vi "USB2XXXGPIOTest.vi"() -> ()   [LabVIEW 2010]
uses:
  PublicFiles/USB2XXX.dll
panel:
  out "P15":bool
  out "P14":bool
  out "P13":bool
  out "P12":bool
  out "P11":bool
  out "P10":bool
  out "P9":bool
  out "P8":bool
  in  "P7":bool
  in  "P6":bool
  in  "P5":bool
  in  "P4":bool
  in  "P3":bool
  in  "P2":bool
  in  "P1":bool
  in  "P0":bool
  in  "Device Index":i32(ring) items=["0", "1", "2", "3", "4", "5"]
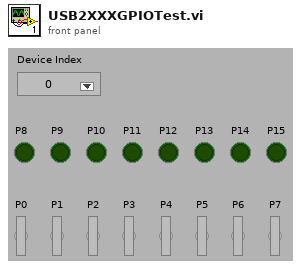
[diagram p1: front panel]
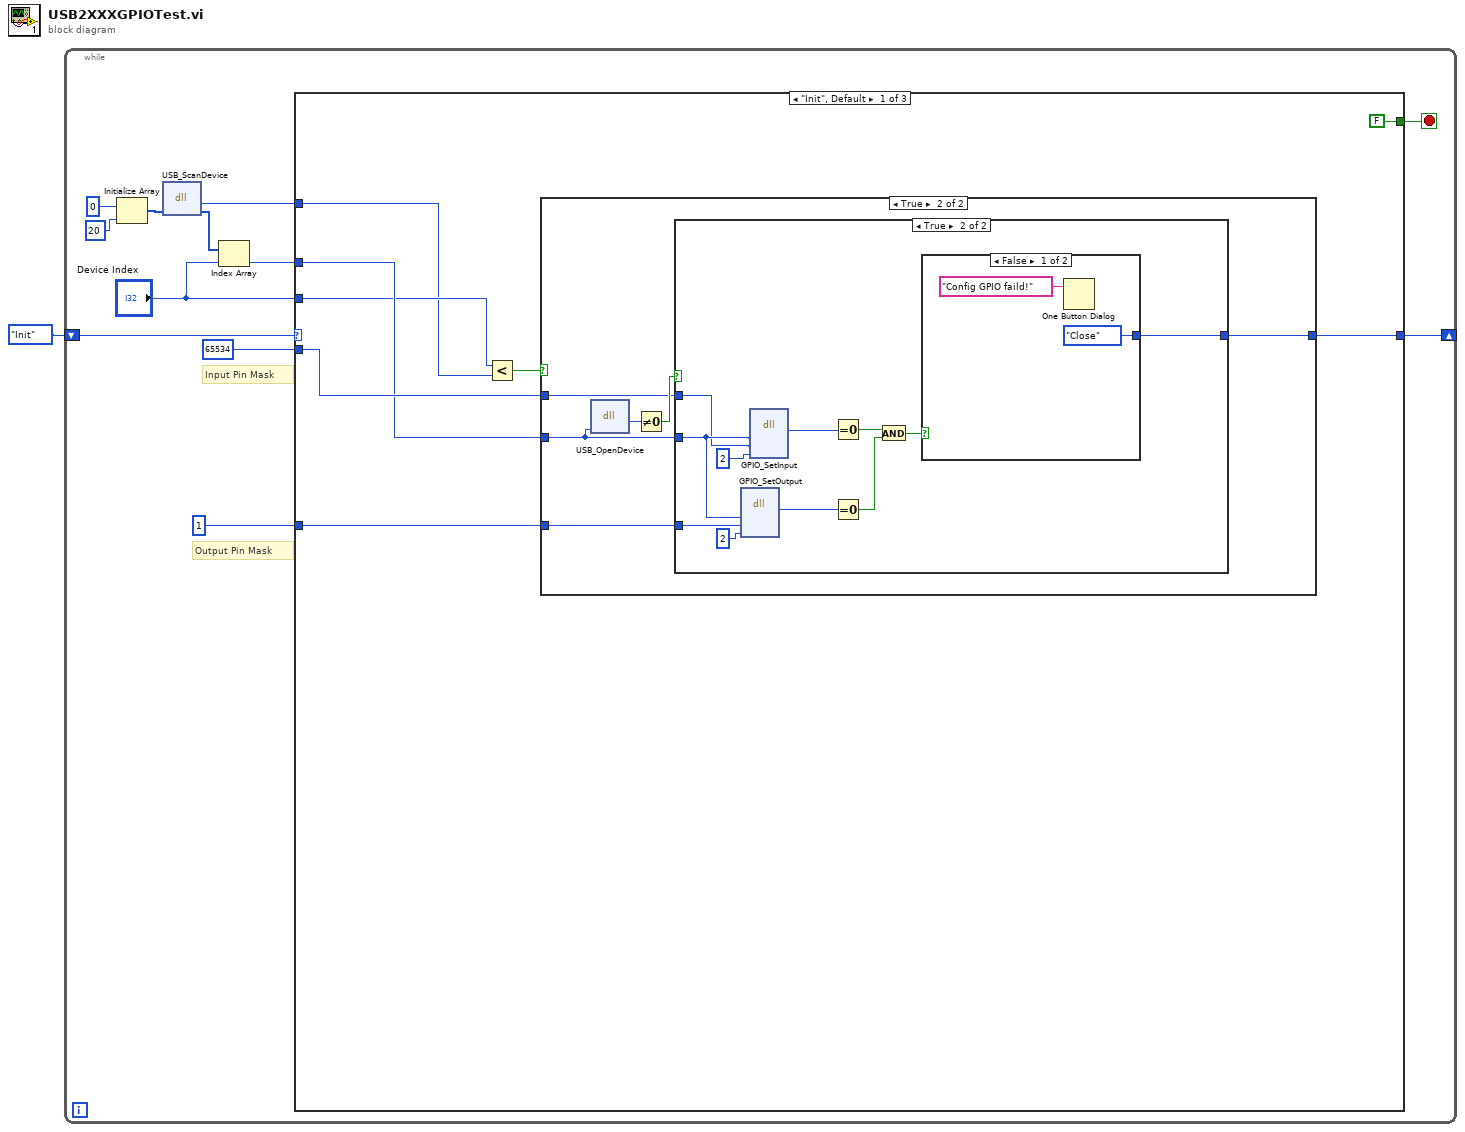
[diagram p0: block diagram]
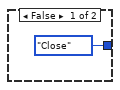
[diagram p2: hidden frame]
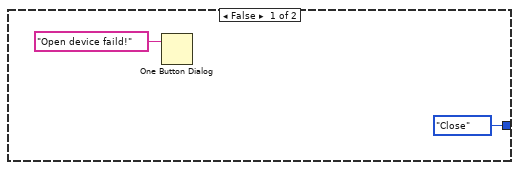
[diagram p3: hidden frame]
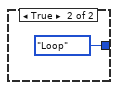
[diagram p4: hidden frame]
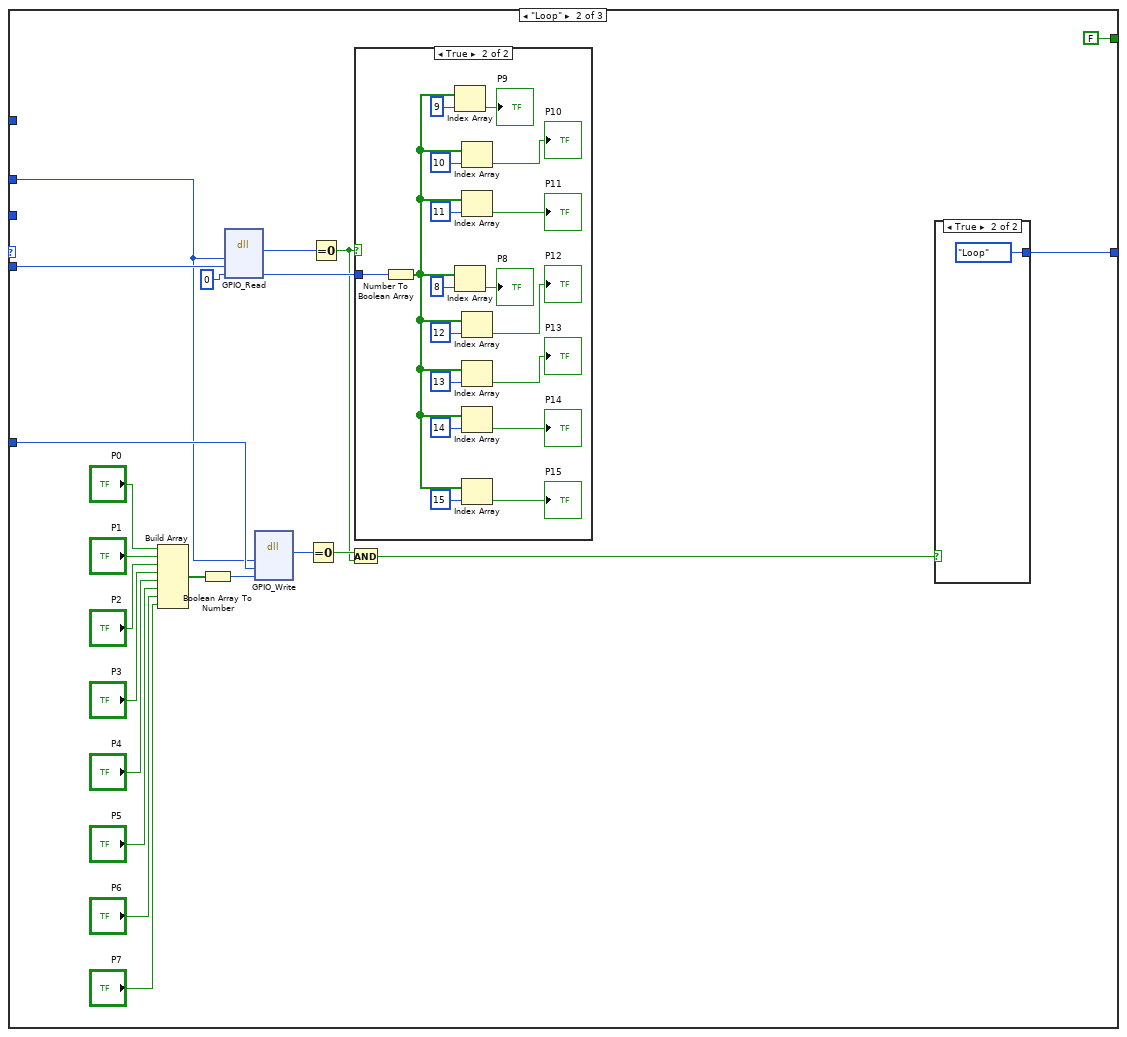
[diagram p5: hidden frame]
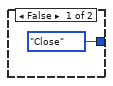
[diagram p6: hidden frame]
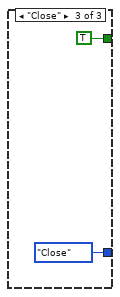
[diagram p8: hidden frame]
diagram:
  n1 = while {
    shift-right: [w12] -> _
    shift-left: enum16{"Init", "Loop", "Close"}."Init" ("Enum") -> [w13]
    stop <- w11 stop-if-true
    # "Output Pin Mask"
    # "Input Pin Mask"
    n2 = Initialize Array(0, 20 ("dimension size")) -> (w8:i32[])
    n3 = dll-call lib="E:/OtherWork/STM32/USB2XXX_Example/trunk/Labview/PublicFiles/USB2XXX.*" fn="USB_ScanDevice"("pDevNum"=w8) -> ("return type"=w4:i32, "pDevNum"=w5:i32[])  [unwired: 3 in, 2 out]
    n4 = Index Array(array=w5, index="Device Index") -> (element=w3:i32)
    n5 = case shown="\"Init\", Default" w13 {
      tunnel: [w20 w46 enum16{"Init", "Loop", "Close"}."Close" ("Enum")] -> w12
      tunnel: u32 65534 -> [w17 w54 _]
      tunnel: [FALSE FALSE TRUE] -> w11
      tunnel: u32 1 -> [w18 w56 _]
      tunnel: w4 -> [w14 _ _]
      tunnel: w3 -> [w16 w45 _]
      tunnel: "Device Index" -> [w15 _ _]
      frame "Init", Default {
        n6 = Less?(x=w15, y=w14) -> (x < y?=w21:bool)
        n7 = case shown="True" w21 {
          tunnel: w16 -> [_ w26]
          tunnel: [enum16{"Init", "Loop", "Close"}."Close" ("Enum") w25] -> w20
          tunnel: w18 -> [_ w24]
          tunnel: w17 -> [_ w23]
          frame False {
          }
          frame True {
            n8 = dll-call lib="E:/OtherWork/STM32/USB2XXX_Example/trunk/Labview/PublicFiles/USB2XXX.*" fn="USB_OpenDevice"("DevIndex"=w26) -> (w28:u8)  [unwired: 4 in, 2 out]
            n9 = Not Equal To 0?(x=w28) -> (x != 0?=w27:bool)
            n10 = case shown="True" w27 {
              tunnel: w26 -> [_ w34]
              tunnel: [enum16{"Init", "Loop", "Close"}."Close" ("Enum") w41] -> w25
              tunnel: w24 -> [_ w40]
              tunnel: w23 -> [_ w33]
              frame False {
                n11 = One Button Dialog(message="Open device faild!") -> ()  [unwired: 1 in, 1 out]
              }
              frame True {
                n12 = dll-call lib="E:/OtherWork/STM32/USB2XXX_Example/trunk/Labview/PublicFiles/USB2XXX.*" fn="GPIO_SetOutput"("DevIndex"=w34, "PinMask"=w40, "PuPd"=u8 2) -> (w38:i32)  [unwired: 6 in, 2 out]
                n13 = dll-call lib="E:/OtherWork/STM32/USB2XXX_Example/trunk/Labview/PublicFiles/USB2XXX.*" fn="GPIO_SetInput"("DevHandle"=w34, "PinMask"=w33, "PuPd"=u8 2) -> (w31:i32)  [unwired: 6 in, 2 out]
                n14 = Equal To 0?(x=w31) -> (x = 0?=w37:bool)
                n15 = Equal To 0?(x=w38) -> (x = 0?=w36:bool)
                n16 = And(x=w37, y=w36) -> (x .and. y?=w35:bool)
                n17 = case shown="False" w35 {
                  tunnel: [enum16{"Init", "Loop", "Close"}."Close" ("Enum") enum16{"Init", "Loop", "Close"}."Loop" ("Enum")] -> w41
                  frame False {
                    n18 = One Button Dialog(message="Config GPIO faild!") -> ()  [unwired: 1 in, 1 out]
                  }
                  frame True {
                  }
                }
              }
            }
          }
        }
      }
      frame "Loop" {
        n19 = Build Array("P0", "P1", "P2", "P3", "P4", "P5", "P6", "P7") -> (w57:bool[])
        n20 = Boolean Array To Number(Boolean array=w57) -> (number=w55:u32)
        n21 = dll-call lib="E:/OtherWork/STM32/USB2XXX_Example/trunk/Labview/PublicFiles/USB2XXX.*" fn="GPIO_Read"("DevIndex"=w45, "PinMask"=w54, "pPinValue"=u32 0) -> (w52:i32, "pPinValue"=w51:u32)  [unwired: 5 in, 2 out]
        n22 = dll-call lib="E:/OtherWork/STM32/USB2XXX_Example/trunk/Labview/PublicFiles/USB2XXX.*" fn="GPIO_Write"("DevIndex"=w45, "PinMask"=w56, "PinValue"=w55) -> (w50:i32)  [unwired: 6 in, 2 out]
        n23 = Equal To 0?(x=w50) -> (x = 0?=w49:bool)
        n24 = Equal To 0?(x=w52) -> (x = 0?=w48:bool)
        n25 = And(x=w49, y=w48) -> (x .and. y?=w47:bool)
        n26 = case shown="True" w48 {
          tunnel: w51 -> [_ w86]
          frame False {
          }
          frame True {
            n27 = Number To Boolean Array(number=w86) -> (Boolean array=w76:bool[])
            n28 = Index Array(array=w76, index=9) -> (element=→"P9":bool)
            n29 = Index Array(array=w76, index=8) -> (element=→"P8":bool)
            n30 = Index Array(array=w76, index=10) -> (element=→"P10":bool)
            n31 = Index Array(array=w76, index=11) -> (element=→"P11":bool)
            n32 = Index Array(array=w76, index=12) -> (element=→"P12":bool)
            n33 = Index Array(array=w76, index=13) -> (element=→"P13":bool)
            n34 = Index Array(array=w76, index=14) -> (element=→"P14":bool)
            n35 = Index Array(array=w76, index=15) -> (element=→"P15":bool)
          }
        }
        n36 = case shown="True" w47 {
          tunnel: [enum16{"Init", "Loop", "Close"}."Close" ("Enum") enum16{"Init", "Loop", "Close"}."Loop" ("Enum")] -> w46
          frame False {
          }
          frame True {
          }
        }
      }
      frame "Close" {
      }
    }
  }
